vi "XNET Read (State J1939 Comm).vi"(0 "session in":refnum<k21>, 11 "error in (no error)":errorcluster) -> (4 "session out":refnum<k21>, 6 "J1939 comm":T1 {"fault code" format="%08x"}, 15 "error out":errorcluster)   [LabVIEW 2018]
doc: "Reads the state of J1939 communication using an XNET session."
uses:
  XNET J1939 Comm.ctl
  nixlvapi.dll
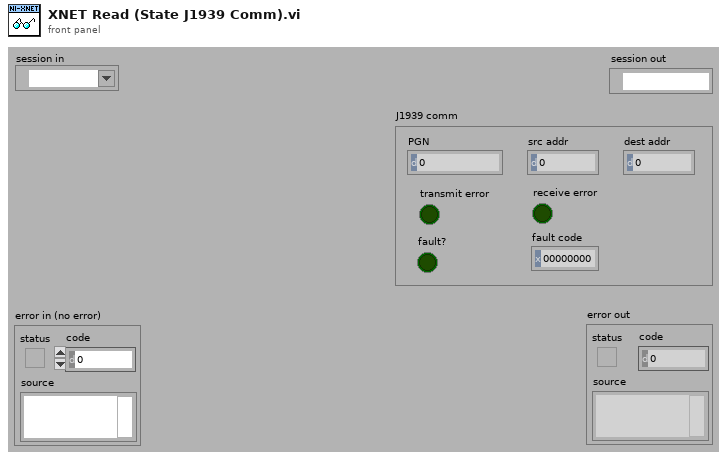
[diagram p1: front panel]
types:
  T1 = typedef "XNET J1939 Comm.ctl" = cluster{"fault code":i32, "fault?":bool, "PGN":u32, "src addr":u8, "dest addr":u8, "transmit error":bool, "receive error":bool}
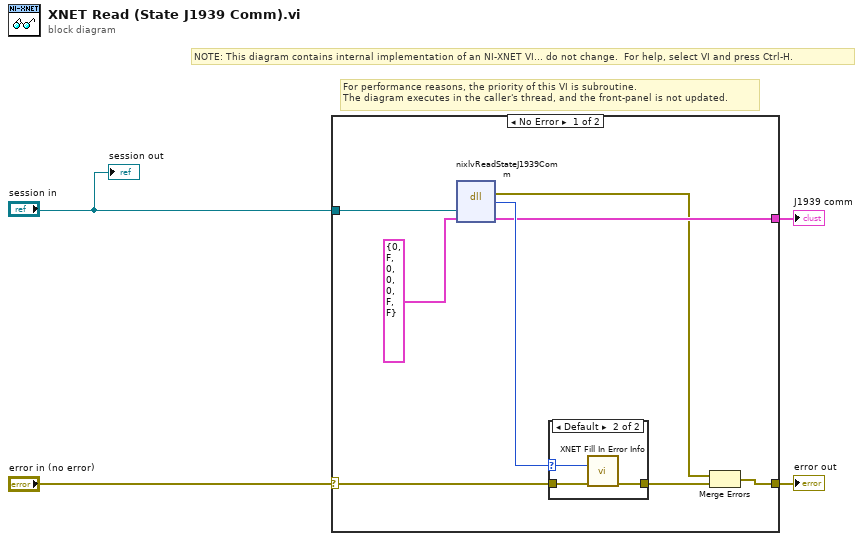
[diagram p0: block diagram]
diagram:
  # "For performance reasons, the priority of this VI is subroutine.\nThe diagram executes in the caller's thread, and the front-panel is not updated."
  # "NOTE: This diagram contains internal implementation of an NI-XNET VI... do not change.  For help, select VI and press Ctrl-H."
  n1 = case shown="No Error" "error in (no error)" {
    selector: "error in (no error)" -> [w11 w17]
    tunnel: "session in" -> [w12 _]
    tunnel: [w6 w17] -> w4
    tunnel: [w7 _] -> w1
    frame No Error {
      n2 = dll-call lib="nixlvapi.*" fn="nixlvReadStateJ1939Comm"("sessionRef"=w12, "J1939Comm"=T1 {"fault code"=0, "fault?"=FALSE, "PGN"=0, "src addr"=0, "dest addr"=0, "transmit error"=FALSE, "receive error"=FALSE} ("J1939 comm")) -> (error out=w5:errorcluster, "return type"=w9:i32, "J1939Comm"=w7:T1)  [unwired: 3 in, 2 out]
      n3 = case shown="Default" w9 {
        selector: w9 -> [_ w14]
        tunnel: w11 -> [w13 w15]
        tunnel: [w13 w16] -> w10
        frame 0 {
        }
        frame Default {
          n4 = call "XNET Fill In Error Info.vi"("status code"=w14, "error in"=w15) -> ("error out"=w16:errorcluster)  [unwired: 13 out]
        }
      }
      n5 = Merge Errors(w5, w10) -> (w6:errorcluster)
    }
    frame Error {
    }
  }
  "error out" <- w4
  "J1939 comm" <- w1
  "session out" <- "session in"
